vi "SourceOpenCOM.vi"(3 "COM Port in":refnum<visa-resource-name>, 9 "error in (no error)":errorcluster) -> (0 "COM Port out":refnum<visa-resource-name>, 6 "error out":errorcluster)   [LabVIEW 2009]
uses:
  <vilib>/Instr/_visa.llb/VISA Configure Serial Port (Serial Instr).vi
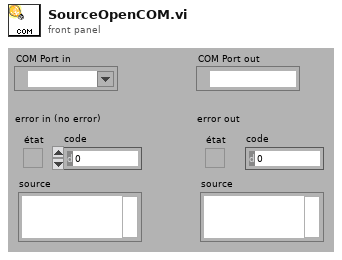
[diagram p1: front panel]
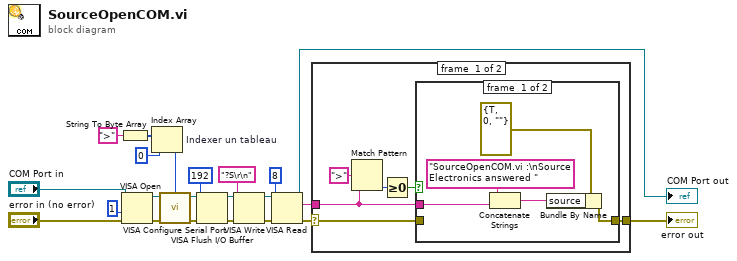
[diagram p0: block diagram]
diagram:
  n1 = String To Byte Array(string=">") -> (unsigned byte array=w8:u8[])
  n2 = VISA Open(access mode=u32 1 ("mode d'accès"), error in (no error)="error in (no error)", VISA resource name="COM Port in") -> (VISA resource name=w4:refnum<visa-resource-name>, error out=w3:errorcluster)  [unwired: 2 out]
  n3 = Index Array "Indexer un tableau"(array=w8, index=0 ("indice")) -> (element=w6:u8)
  n4 = call-poly "VISA Configure Serial Port"("VISA resource name"=w4, "termination char\n(0xA = '\\n' = LF)"=w6, "error in (no error)"=w3) -> ("VISA resource name out"=w14:refnum<visa-resource-name>, "error out"=w13:errorcluster)  [unwired: 4 in, 7 out]
  n5 = VISA Flush I/O Buffer(VISA resource name=w14, mask (16)=u16 192 ("masque (16)"), error in (no error)=w13) -> (VISA resource name out=w15:refnum<visa-resource-name>, error out=w16:errorcluster)
  n6 = VISA Write(VISA resource name=w15, write buffer="?S\r\n" ("buffer à écrire"), error in (no error)=w16) -> (VISA resource name out=w10:refnum<visa-resource-name>, error out=w11:errorcluster)  [unwired: 1 out]
  n7 = VISA Read(VISA resource name=w10, byte count=u32 8 ("nombre d'octets (0)"), error in (no error)=w11) -> (VISA resource name out=→"COM Port out":refnum<visa-resource-name>, read buffer=w22:string, error out=w21:errorcluster)  [unwired: 1 out]
  n8 = case shown="No Error" w21 {
    selector: w21 -> [w23 w35]
    tunnel: w22 -> [w25 _]
    tunnel: [w24 w35] -> w2
    frame #0 {
      n9 = Match Pattern(string=w25, regular expression=">" ("expression")) -> (offset past match=w27:i32)  [unwired: 4 out]
      n10 = Greater Or Equal To 0?(x=w27) -> (x >= 0?=w26:bool)
      n11 = case shown="True" w26 {
        tunnel: w23 -> [_ w34]
        tunnel: [w32 w34] -> w24
        tunnel: w25 -> [w33 _]
        frame #0 {
          n12 = Concatenate Strings("SourceOpenCOM.vi :\nSource Electronics answered " ("source"), w33) -> (w30:string)
          n13 = Bundle By Name(cluster=errorcluster {"status"=TRUE, "code"=0, "source"=""} ("error out"), "source"=w30) -> (w32:errorcluster)
        }
        frame #1 {
        }
      }
    }
    frame #1 {
    }
  }
  "error out" <- w2
